vi "VISAInit.vi"(8 "Use Stage?":bool, 9 "Use DM?":bool, 10 "DM Resource Name":refnum<visa-resource-name> caption="resource name", 11 "Stage Resource Name":refnum<visa-resource-name>) -> (0 "error out":errorcluster, 2 "DM Handle":refnum<visa-resource-name> caption="instrument handle out", 3 "Stage Resource":refnum<visa-resource-name>)   [LabVIEW 2018]
uses:
  <vilib>/Instr/_visa.llb/VISA Configure Serial Port (Instr).vi
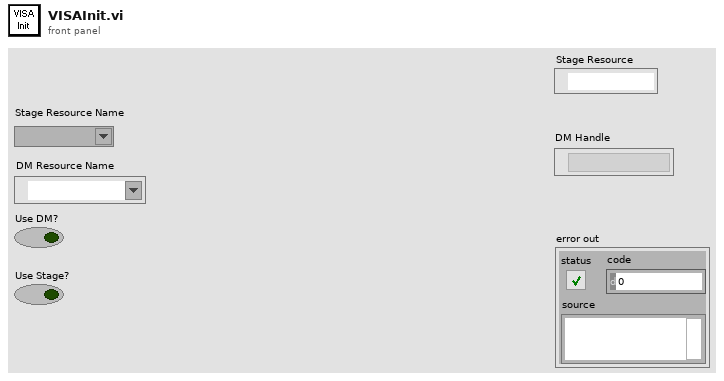
[diagram p1: front panel]
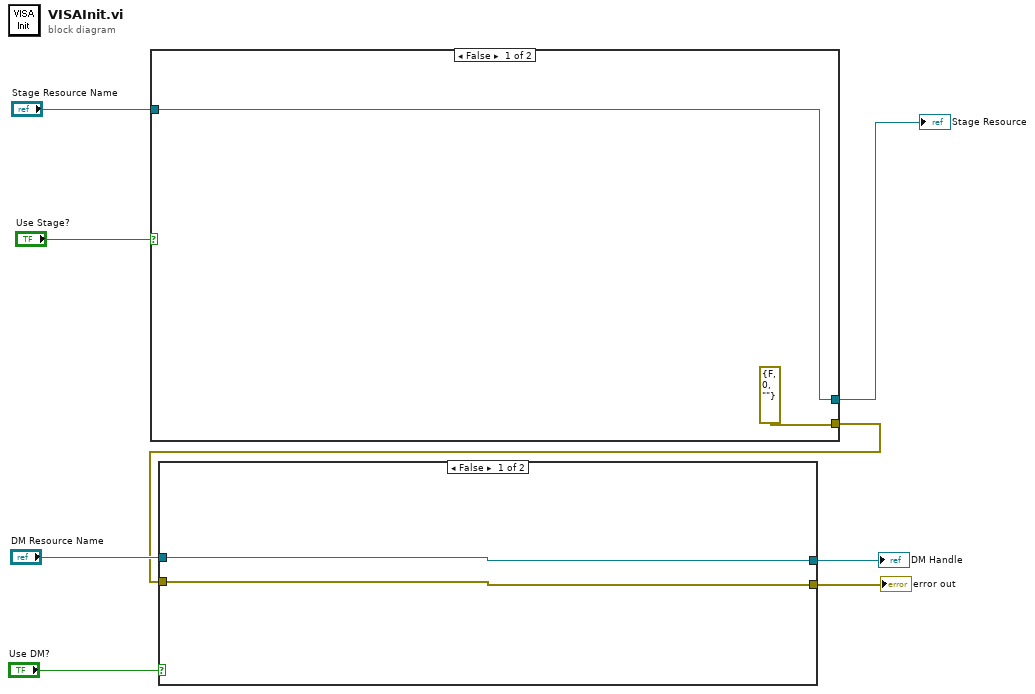
[diagram p0: block diagram]
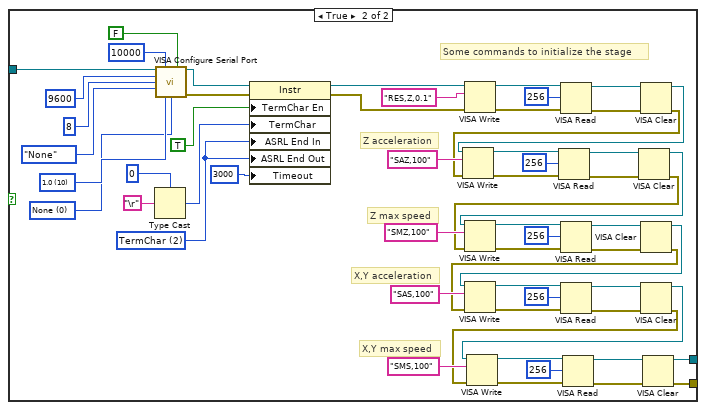
[diagram p2: hidden frame]
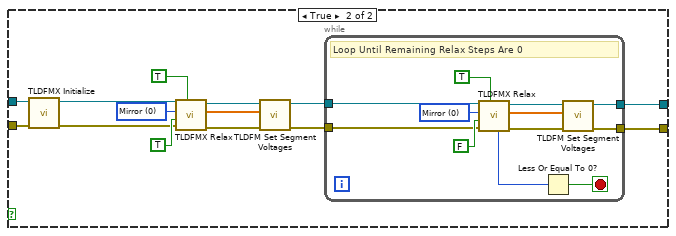
[diagram p3: hidden frame]
diagram:
  n1 = case shown="False" "Use Stage?" {
    tunnel: "Stage Resource Name" -> [w9 w53]
    tunnel: [w9 w12] -> w7
    tunnel: [errorcluster {"status"=FALSE, "code"=0, "source"=""} ("error out") w11] -> w5
    frame False {
    }
    frame True {
      w54 = u16 2 items=["None", "Last Bit", "TermChar"] ("Serial Settings:End Mode for Reads")
      w62 = u16 0 items=["None", "XON/XOFF", "RTS/CTS", "XON/XOFF & RTS/CTS", "DTR/DSR", "XON/XOFF & DTR/DSR"] ("flow control (0:none)")
      w63 = u16 10 items=["1.0"=10, "1.5"=15, "2.0"=20] ("stop bits (10: 1 bit)")
      # "Z max speed"
      # "X,Y max speed"
      # "X,Y acceleration"
      # "Z acceleration"
      # "Some commands to initialize the stage"
      n2 = Type Cast(type=u8 0 ("Message Based Settings:Termination Character"), x="\r") -> (*(type *) &x=w59:u8)
      n3 = call-poly "VISA Configure Serial Port"("VISA resource name"=w53, "timeout (10sec)"=u32 10000, "Enable Termination\nChar (T)"=FALSE ("Enable Termination\nChar (T)"), "baud rate (9600)"=u32 9600, "data bits (8)"=u16 8, "parity (0:none)"=enum16{"None", "Odd", "Even", "Mark", "Space"}."None", "stop bits (10: 1 bit)"=w63, "flow control (0:none)"=w62) -> ("VISA resource name out"=w58:refnum<visa-resource-name>, "error out"=w57:errorcluster)  [unwired: 6 in]
      n4 = property class="Instr"(reference=w58, error in=w57, "TermChar En"=TRUE ("Message Based Settings:Termination Character Enable"), "TermChar"=w59, "ASRL End In"=w54, "ASRL End Out"=w54, "Timeout"=u32 3000 ("General Settings:Timeout Value")) -> (reference out=w47:refnum<visa-resource-name>, error out=w46:errorcluster)
      n5 = VISA Write(VISA resource name=w47, write buffer="RES,Z,0.1" ("string"), error in (no error)=w46) -> (VISA resource name out=w49:refnum<visa-resource-name>, error out=w50:errorcluster)  [unwired: 1 out]
      n6 = VISA Read(VISA resource name=w49, byte count=u32 256, error in (no error)=w50) -> (VISA resource name out=w52:refnum<visa-resource-name>, error out=w51:errorcluster)  [unwired: 2 out]
      n7 = VISA Clear(VISA resource name=w52, error in (no error)=w51) -> (VISA resource name out=w18:refnum<visa-resource-name>, error out=w20:errorcluster)
      n8 = VISA Write(VISA resource name=w18, write buffer="SAZ,100" ("string"), error in (no error)=w20) -> (VISA resource name out=w41:refnum<visa-resource-name>, error out=w42:errorcluster)  [unwired: 1 out]
      n9 = VISA Read(VISA resource name=w41, byte count=u32 256, error in (no error)=w42) -> (VISA resource name out=w44:refnum<visa-resource-name>, error out=w43:errorcluster)  [unwired: 2 out]
      n10 = VISA Clear(VISA resource name=w44, error in (no error)=w43) -> (VISA resource name out=w17:refnum<visa-resource-name>, error out=w19:errorcluster)
      n11 = VISA Write(VISA resource name=w17, write buffer="SMZ,100" ("string"), error in (no error)=w19) -> (VISA resource name out=w36:refnum<visa-resource-name>, error out=w35:errorcluster)  [unwired: 1 out]
      n12 = VISA Read(VISA resource name=w36, byte count=u32 256, error in (no error)=w35) -> (VISA resource name out=w33:refnum<visa-resource-name>, error out=w34:errorcluster)  [unwired: 2 out]
      n13 = VISA Clear(VISA resource name=w33, error in (no error)=w34) -> (VISA resource name out=w15:refnum<visa-resource-name>, error out=w16:errorcluster)
      n14 = VISA Write(VISA resource name=w15, write buffer="SAS,100" ("string"), error in (no error)=w16) -> (VISA resource name out=w29:refnum<visa-resource-name>, error out=w30:errorcluster)  [unwired: 1 out]
      n15 = VISA Read(VISA resource name=w29, byte count=u32 256, error in (no error)=w30) -> (VISA resource name out=w32:refnum<visa-resource-name>, error out=w31:errorcluster)  [unwired: 2 out]
      n16 = VISA Clear(VISA resource name=w32, error in (no error)=w31) -> (VISA resource name out=w14:refnum<visa-resource-name>, error out=w13:errorcluster)
      n17 = VISA Write(VISA resource name=w14, write buffer="SMS,100" ("string"), error in (no error)=w13) -> (VISA resource name out=w24:refnum<visa-resource-name>, error out=w23:errorcluster)  [unwired: 1 out]
      n18 = VISA Read(VISA resource name=w24, byte count=u32 256, error in (no error)=w23) -> (VISA resource name out=w21:refnum<visa-resource-name>, error out=w22:errorcluster)  [unwired: 2 out]
      n19 = VISA Clear(VISA resource name=w21, error in (no error)=w22) -> (VISA resource name out=w12:refnum<visa-resource-name>, error out=w11:errorcluster)
    }
  }
  "Stage Resource" <- w7
  n20 = case shown="False" "Use DM?" {
    tunnel: "DM Resource Name" -> [w69 w84]
    tunnel: w5 -> [w70 w83]
    tunnel: [w69 w72] -> w4
    tunnel: [w70 w71] -> w3
    frame False {
    }
    frame True {
      w75 = u32 0 items=["Mirror", "Arms", "Mirror + Arms"] ("Device Part (Mirror)")
      n21 = call "TLDFMX Initialize.vi"("error in (no error)"=w83, "resource name"=w84) -> ("error out"=w73:errorcluster, "instrument handle out"=w74:refnum<visa-resource-name>)  [unwired: 8 in]
      n22 = call "TLDFMX Relax.vi"("Reload (1)"=TRUE, "error in (no error)"=w73, "Is First Step (0)"=TRUE, "Device Part (Mirror)"=w75, "instrument handle"=w74) -> ("error out"=w79:errorcluster, "Relax Pattern Mirror (0)"=w80:dbl[], "instrument handle out"=w78:refnum<visa-resource-name>)  [unwired: 2 in, 2 out]
      n23 = call "TLDFM Set Segment Voltages.vi"("error in (no error)"=w79, "Segment Voltages"=w80, "instrument handle"=w78) -> ("error out"=w82:errorcluster, "instrument handle out"=w81:refnum<visa-resource-name>)  [unwired: 7 in]
      n24 = while {
        tunnel: w81 -> [w90]
        tunnel: w82 -> [w89]
        tunnel: [w86] -> w72
        tunnel: [w85] -> w71
        stop <- w87 stop-if-true
        w91 = u32 0 items=["Mirror", "Arms", "Mirror + Arms"] ("Device Part (Mirror)")
        # "Loop Until Remaining Relax Steps Are 0"
        n25 = call "TLDFMX Relax.vi"("Reload (1)"=TRUE, "error in (no error)"=w89, "Is First Step (0)"=FALSE, "Device Part (Mirror)"=w91, "instrument handle"=w90) -> ("error out"=w95:errorcluster, "Relax Pattern Mirror (0)"=w96:dbl[], "instrument handle out"=w94:refnum<visa-resource-name>, "Remaining Steps"=w88:i32)  [unwired: 2 in, 1 out]
        n26 = Less Or Equal To 0?(x=w88) -> (x <= 0?=w87:bool)
        n27 = call "TLDFM Set Segment Voltages.vi"("error in (no error)"=w95, "Segment Voltages"=w96, "instrument handle"=w94) -> ("error out"=w85:errorcluster, "instrument handle out"=w86:refnum<visa-resource-name>)  [unwired: 7 in]
      }
    }
  }
  "error out" <- w3
  "DM Handle" <- w4
